vi "NI VeriStand - FPGA PWM In.vi"(9 "Time Out":u32=40000, 11 "Value":bool) -> (0 "High time":u32, 2 "Low Time":u32)   [LabVIEW 2020, in "NI_VS FPGA Support.lvlib"]
uses:
  <vilib>/NI VeriStand/FPGA/NI_VS FPGA Support.lvlib
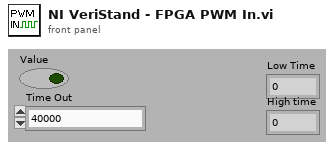
[diagram p1: front panel]
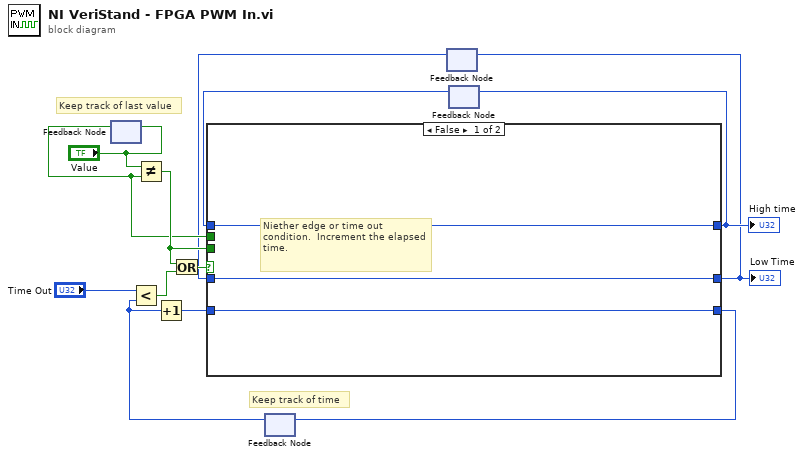
[diagram p0: block diagram]
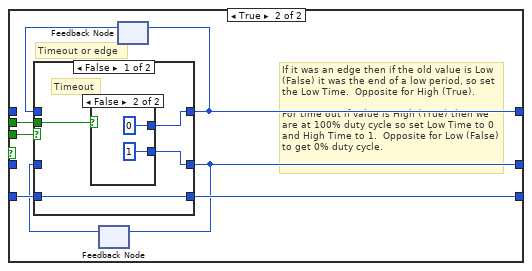
[diagram p2: hidden frame]
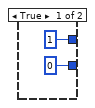
[diagram p3: hidden frame]
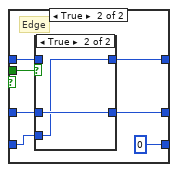
[diagram p4: hidden frame]
diagram:
  # "Keep track of last value"
  # "Keep track of time"
  n1 = feedback-in #1("Value") -> ()
  n2 = feedback #1() -> (w5:bool)  [unwired: 1 out]
  n3 = Not Equal?(x="Value", y=w5) -> (x != y?=w10:bool)
  n4 = feedback #2() -> (w6:u32)  [unwired: 1 out]
  n5 = Less?(x="Time Out", y=w6) -> (x < y?=w12:bool)
  n6 = Increment(x=w6) -> (x+1=w7:u32)
  n7 = Or(x=w10, y=w12) -> (x .or. y?=w11:bool)
  n8 = feedback #3() -> (w1:u32)  [unwired: 1 out]
  n9 = feedback #4() -> (w2:u32)  [unwired: 1 out]
  n10 = case shown="False" w11 {
    tunnel: w5 -> [_ w21]
    tunnel: w10 -> [_ w24]
    tunnel: w7 -> [w16 w23]
    tunnel: [w16 w22] -> w9
    tunnel: [w14 w18] -> w3
    tunnel: [w15 w17] -> w4
    tunnel: w2 -> [w15 _]
    tunnel: w1 -> [w14 _]
    frame False {
      # "Niether edge or time out condition.  Increment the elapsed time."
    }
    frame True {
      # "If it was an edge then if the old value is Low (False) it was the end of a low period, so set the Low Time.  Opposite for High (True).\n\nFor time out if value is High (True) then we are at 100% duty cycle so set Low Time to 0 and High Time to 1.  Opposite for Low (False) to get 0% duty cycle."
      # "Timeout or edge"
      n11 = feedback #5() -> (w20:u32)  [unwired: 1 out]
      n12 = feedback #6() -> (w19:u32)  [unwired: 1 out]
      n13 = case shown="False" w24 {
        tunnel: w23 -> [w28 w36]
        tunnel: [w28 u32 0 ("Time")] -> w22
        tunnel: w21 -> [w27 w38]
        tunnel: [w25 w37] -> w18
        tunnel: w20 -> [_ w35]
        tunnel: [w26 w34] -> w17
        tunnel: w19 -> [_ w33]
        frame False {
          # "Timeout"
          n14 = case shown="False" w27 {
            tunnel: [u32 1 u32 0] -> w26
            tunnel: [u32 0 u32 1] -> w25
            frame True {
            }
            frame False {
            }
          }
        }
        frame True {
          # "Edge"
          n15 = case shown="True" w38 {
            tunnel: [w41 w43] -> w37
            tunnel: w36 -> [w41 w42]
            tunnel: w35 -> [_ w43]
            tunnel: [w40 w42] -> w34
            tunnel: w33 -> [w40 _]
            frame False {
            }
            frame True {
            }
          }
        }
      }
      n16 = feedback-in #5(w18) -> ()
      n17 = feedback-in #6(w17) -> ()
    }
  }
  "High time" <- w4
  "Low Time" <- w3
  n18 = feedback-in #2(w9) -> ()
  n19 = feedback-in #3(w3) -> ()
  n20 = feedback-in #4(w4) -> ()
